vi "DataTreeCtrlFM updComment.vi"(7 "newItemNames":string[](array[string]), 8 "error in (no error)":errorcluster, 11 "DataTreeCtrl in":refnum<class "DataTreeCtrl.lvclass">) -> (0 "error out":errorcluster, 3 "DataTreeCtrl out":refnum<class "DataTreeCtrl.lvclass">)   [LabVIEW 2018, in "DataTreeCtrl.lvclass"]
uses:
  DataTreeCtrl.lvclass
  ctl/FMstateMachineEnum.ctl
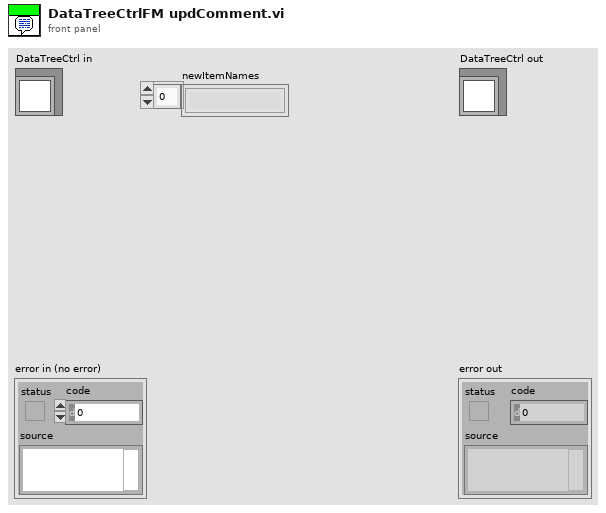
[diagram p1: front panel]
types:
  T1 = typedef "FMstateMachineEnum.ctl" = enum16{"none", "init", "openTDMS", "closeTDMS", "getDataList", "getDataInfo", "getTimeStamp", "getCurrPath", "getRemark", "overwriteRemark", "readData", "deleteData", "moveData"}
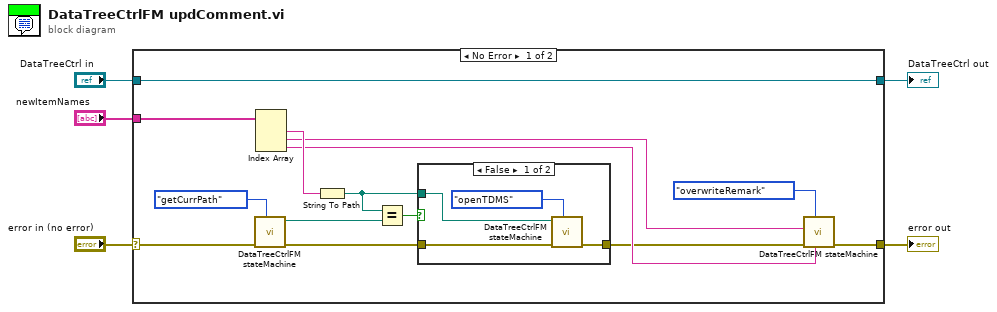
[diagram p0: block diagram]
diagram:
  n1 = case shown="No Error" "error in (no error)" {
    selector: "error in (no error)" -> [w16 w26]
    tunnel: [w14 w26] -> w4
    tunnel: [w19 w25] -> w2
    tunnel: "DataTreeCtrl in" -> [w19 w25]
    tunnel: "newItemNames" -> [w7 _]
    frame No Error {
      n2 = call "DataTreeCtrlFM stateMachine.vi"("Func"=FMstateMachineEnum."getCurrPath", "error in (no error)"=w16) -> ("error out"=w17:errorcluster, "tdmsFilePath out"=w15:path)  [unwired: 4 in, 4 out]
      n3 = Index Array(array=w7) -> (element #1=w11:string, element #2=w9:string, element #3=w10:string)  [unwired: 3 in]
      n4 = String To Path(string=w11) -> (path=w12:path)
      n5 = Equal?(x=w12, y=w15) -> (x = y?=w13:bool)
      n6 = case shown="False" w13 {
        tunnel: w17 -> [w21 w24]
        tunnel: [w20 w24] -> w8
        tunnel: w12 -> [w22 _]
        frame False {
          n7 = call "DataTreeCtrlFM stateMachine.vi"("Func"=FMstateMachineEnum."openTDMS", "error in (no error)"=w21, "tdmsFilePath in"=w22) -> ("error out"=w20:errorcluster)  [unwired: 3 in, 5 out]
        }
        frame True {
        }
      }
      n8 = call "DataTreeCtrlFM stateMachine.vi"("newRemark"=w10, "Func"=FMstateMachineEnum."overwriteRemark", "error in (no error)"=w8, "singleDataName"=w9) -> ("error out"=w14:errorcluster)  [unwired: 2 in, 5 out]
    }
    frame Error {
    }
  }
  "error out" <- w4
  "DataTreeCtrl out" <- w2
